vi "AddedSustainedGaitHeight.vi"(8 "Enum":enum16{"3D", "2D"}(ring)=enum."2D", 10 "ScalingCoef":dbl=1.0, 11 "Averaged Gait":dbl[][](array[numeric])) -> (2 "ScaledGait":dbl[][](array[numeric]), 3 "XY Graph":cluster{"Y":dbl[], "Y":dbl[]}[](graph))   [LabVIEW 2016]
uses:
  <userlib>/_OpenG.lib/array/array.llb/Index 1D Array Elements (DBL)__ogtk.vi
  <vilib>/imath/engines/lvmath2/RunTimeEngine/IndexRead/NIMS V(S).vi
  <instcachedir>/0/NIMS V(S)_0488751826AF41519A22953C041130DC.lvgen/NIMS V(S)_0488751826AF41519A22953C041130DC_000.vi
  <vilib>/imathl/engines/lvmath/Functions/Error Handling/Create Error.vi
  <vilib>/imath/engines/lvmath2/RunTimeEngine/ArithmeticOperatorToken/NIMS_ArithmeticOperator_power(S).vi
  <instcachedir>/0/NIMS_ArithmeticOperator_power(S)_1E6AB98FD36540B9B758A69A385A1B47.lvgen/NIMS_ArithmeticOperator_power(S)_1E6AB98FD36540B9B758A69A385A1B47_015.vi
  <instcachedir>/0/NIMS_ArithmeticOperator_power(S)_1E6AB98FD36540B9B758A69A385A1B47.lvgen/NIMS_ArithmeticOperator_power(S)_1E6AB98FD36540B9B758A69A385A1B47_014.vi
  <vilib>/imath/engines/lvmath2/RunTimeEngine/ErrorHandling/NIMS_Create Error From Enums.vi
  <vilib>/imath/engines/lvmath2/RunTimeEngine/NodeEndStatement/NIMS_NodeEndStatement_Output.vi
  <instcachedir>/0/NIMS_NodeEndStatement_Output_53EC0D466D134D7ABD903AC30B43404B.lvgen/NIMS_NodeEndStatement_Output_53EC0D466D134D7ABD903AC30B43404B_005.vi
  <vilib>/imath/engines/lvmath2/RunTimeEngine/ErrorHandling/NIMS_Finalize Error.vi
panel:
  out "XY Graph 2":cluster{dbl[], "yi":dbl[]}(graph)
  out "XY":cluster{"Mean":dbl[], "Mean":dbl[]}[](array[cluster])
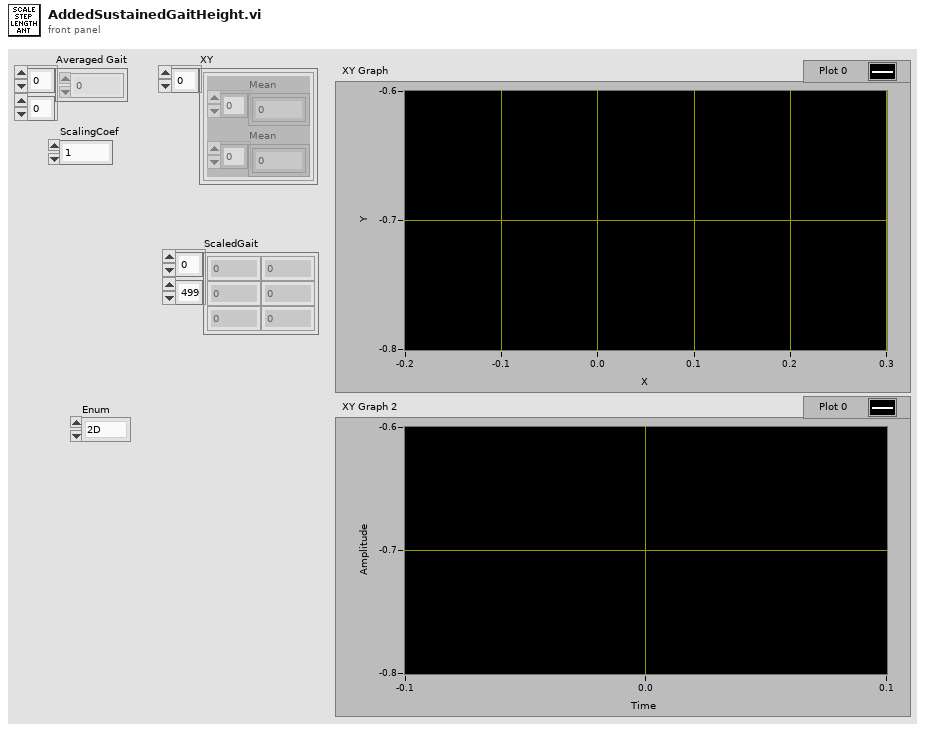
[diagram p1: front panel]
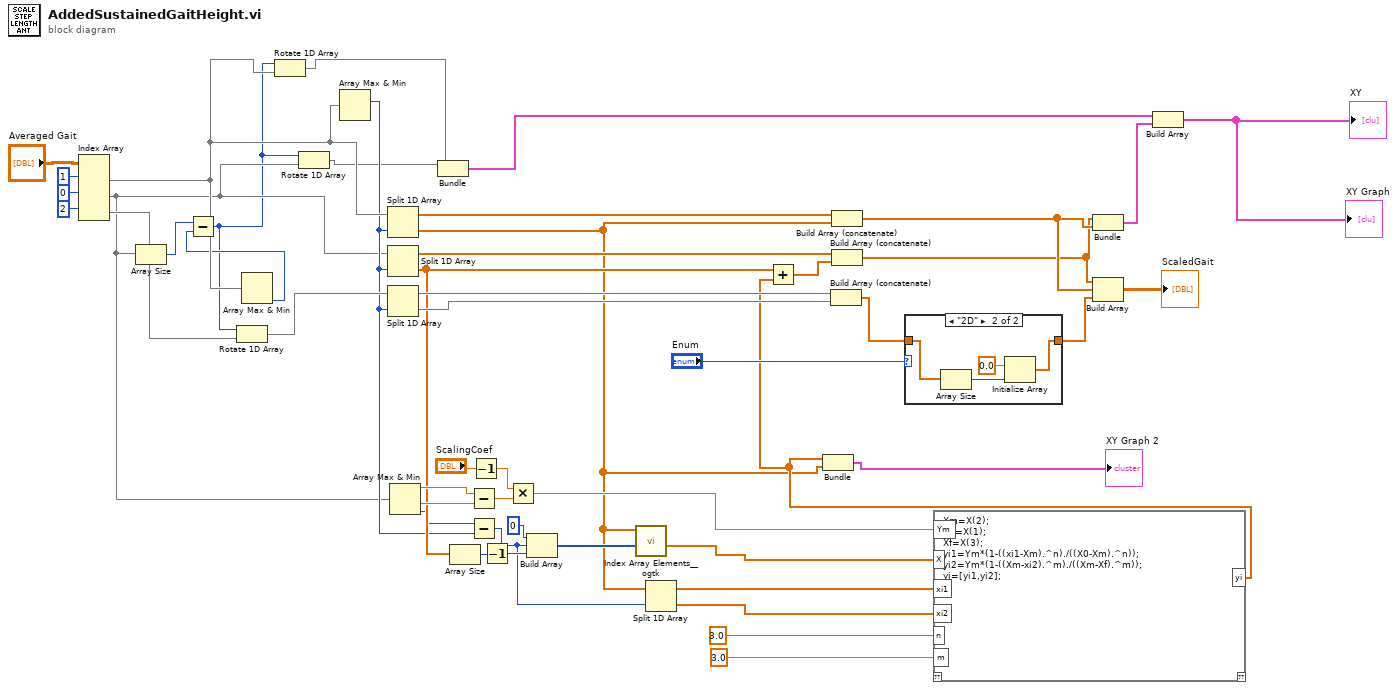
[diagram p0: block diagram]
diagram:
  n1 = Index Array(array="Averaged Gait", index (row) #1=1 ("index (row)"), index (row) #2=0 ("index (row)"), index (row) #3=2 ("index (row)")) -> (element #1=w8:dbl[], element #2=w3:dbl[], element #3=w43:dbl[])  [unwired: 3 in]
  n2 = Array Size(array=w3) -> (size(s)=w45:i32)
  n3 = Array Max & Min(array=w8) -> (min index (indices)=w4:i32)  [unwired: 3 out]
  n4 = Subtract(x=w45, y=w4) -> (x-y=w1:i32)
  n5 = Rotate 1D Array(1:w43, 2:w1) -> (0:w41:dbl[])
  n6 = Rotate 1D Array(1:w8, 2:w1) -> (0:w7:dbl[])
  n7 = Rotate 1D Array(1:w3, 2:w1) -> (0:w2:dbl[])
  n8 = Array Max & Min(array=w8) -> (max index (indices)=w6:i32)  [unwired: 3 out]
  n9 = Split 1D Array(array=w8, index=w6) -> (first subarray=w34:dbl[], second subarray=w11:dbl[])
  n10 = Split 1D Array(array=w3, index=w6) -> (first subarray=w35:dbl[], second subarray=w26:dbl[])
  n11 = Split 1D Array(array=w41, index=w6) -> (first subarray=w33:dbl[], second subarray=w32:dbl[])
  n12 = Array Max & Min(array=w3) -> (max value=w37:dbl, min value=w38:dbl, min index (indices)=w5:i32)  [unwired: 1 out]
  n13 = Bundle(w2, w7) -> (w49:cluster{dbl[], dbl[]})  [unwired: 1 in]
  n14 = Array Size(array=w26) -> (size(s)=w40:i32)
  n15 = Subtract(x=w37, y=w38) -> (x-y=w28:dbl)
  n16 = Subtract(x=w5, y=w6) -> (x-y=w20:i32)
  n17 = Decrement(x="ScalingCoef") -> (x-1=w27:dbl)
  n18 = Decrement(x=w40) -> (x-1=w29:i32)
  n19 = Multiply(x=w27, y=w28) -> (x*y=w23:dbl)
  n20 = Build Array(0 ("element"), w20, w29) -> (w24:i32[])
  n21 = call-poly <userlib>:"Index Array Elements__ogtk.vi"("indices"=w24, "array"=w11) -> ("elements"=w22:dbl[])  [unwired: 9 in]
  n22 = Split 1D Array(array=w11, index=w20) -> (first subarray=w19:dbl[], second subarray=w18:dbl[])
  n23 = Build Array (concatenate)(w33, w32) -> (w14:dbl[])
  n24 = Build Array (concatenate)(w34, w11) -> (w10:dbl[])
  n25 = case shown="\"2D\"" "Enum" {
    tunnel: w14 -> [w50 w54]
    tunnel: [w50 w52] -> w13
    frame "3D", Default {
    }
    frame "2D" {
      n26 = Array Size(array=w54) -> (size(s)=w53:i32)
      n27 = Initialize Array(0.0 ("element"), w53) -> (w52:dbl[])
    }
  }
  n28 = mathscript code="Xm=X(2);\nX0=X(1);\nXf=X(3);\nyi1=Ym*(1-((xi1-Xm).^n)./((X0-Xm).^n));\nyi2=Ym*(1-((Xm-xi2).^m)./((Xm-Xf).^m));\nyi=[yi1,yi2];"("Ym"=w23, "X"=w22, "xi1"=w19, "n"=3.0 ("element"), "xi2"=w18, "m"=3.0 ("element")) -> ("yi"=w12:dbl[])  [unwired: 1 in, 1 out]
  n29 = Add(x=w26, y=w12) -> (x+y=w36:dbl[])
  n30 = Bundle("yi"=w12, w11) -> (→"XY Graph 2":cluster{"yi":dbl[], dbl[]})  [unwired: 1 in]
  n31 = Build Array (concatenate)(w35, w36) -> (w9:dbl[])
  n32 = Bundle(w9, w10) -> (w31:cluster{dbl[], dbl[]})  [unwired: 1 in]
  n33 = Build Array(w9, w10, w13) -> (→"ScaledGait":dbl[][])
  n34 = Build Array(w49, w31) -> (→"XY" →"XY Graph":cluster{dbl[], dbl[]}[])
